vi "getNetworkStreamType.vi"() -> (2 "reader endpoint":refnum<k21>, 3 "writer endpoint":refnum<k21>)   [LabVIEW 2013, in "Connection.NetworkQueue_GOSPL.lvlib" / "Connection.NetworkStream.lvclass"]
uses:
  Connection.NetworkStream/Connection.NetworkStream.lvclass
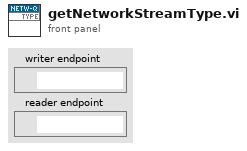
[diagram p1: front panel]
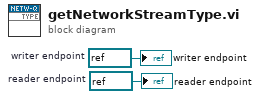
[diagram p0: block diagram]
diagram:
  w1 = refnum<k21> refnum  # reader endpoint
  w2 = refnum<k21> refnum  # writer endpoint
  "writer endpoint" <- w2
  "reader endpoint" <- w1
